vi "Get GUID.vi"(8 "error in (no error)":errorcluster) -> (0 "error out":errorcluster, 3 "GUID":string)   [LabVIEW 2013]
uses:
  <vilib>/registry/registry.llb/Registry RtKey.ctl
  <vilib>/registry/registry.llb/Registry SAM.ctl
  <vilib>/registry/registry.llb/Registry View.ctl
  <vilib>/registry/registry.llb/Read Registry Value Simple STR.vi
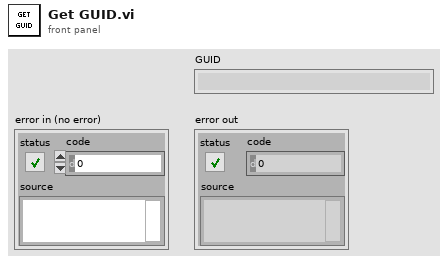
[diagram p1: front panel]
types:
  T1 = typedef "Registry SAM.ctl" = enum32{"KEY_QUERY_VALUE", "KEY_SET_VALUE", "KEY_CREATE_SUB_KEY", "KEY_ENUMERATE_SUB_KEYS", "KEY_NOTIFY", "KEY_CREATE_LINK", "KEY_READ", "KEY_WRITE", "KEY_ALL_ACCESS", "KEY_READ | KEY_WRITE"}
  T2 = typedef "Registry RtKey.ctl" = enum32{"HKEY_CLASSES_ROOT", "HKEY_CURRENT_USER", "HKEY_LOCAL_MACHINE", "HKEY_USERS", "HKEY_PERFORMANCE_DATA", "HKEY_CURRENT_CONFIG", "HKEY_DYN_DATA"}
  T3 = typedef "Registry View.ctl" = u16
  T4 = typedef "Registry refnum.ctl" = refnum<k1>
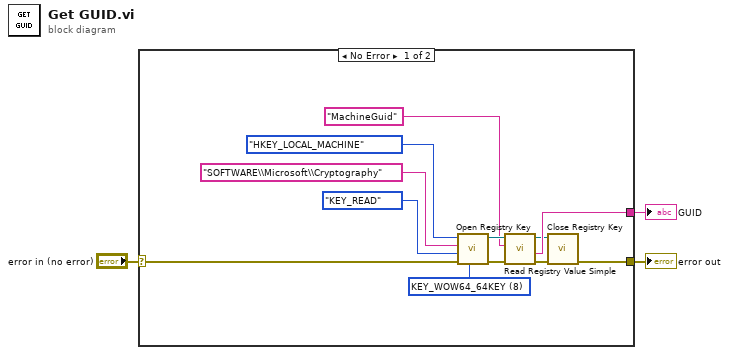
[diagram p0: block diagram]
diagram:
  n1 = case shown="No Error" "error in (no error)" {
    selector: "error in (no error)" -> [w15 w16]
    tunnel: [w14 w16] -> w2
    tunnel: [w13 _] -> w1
    frame No Error {
      w4 = T3 8 items=["Default"=0, "KEY_WOW64_64KEY"=8, "KEY_WOW64_32KEY"=9] ("registry view")
      n2 = call <vilib>:"Open Registry Key.vi"("registry view"=w4, "error in (no error)"=w15, "security access mask (KEY_READ | KEY_WRITE)"=Registry_SAM."KEY_READ", "subkey"="SOFTWARE\\Microsoft\\Cryptography", "root key (HKEY_LOCAL_MACHINE)"=Registry_RtKey."HKEY_LOCAL_MACHINE") -> ("error out"=w8:errorcluster, "refnum out"=w9:T4)  [unwired: 5 in]
      n3 = call-poly <vilib>:"Read Registry Value Simple.vi"("error in (no error)"=w8, "value"="MachineGuid", "refnum"=w9) -> ("error out"=w6:errorcluster, "String/Binary data"=w13:string, "refnum out"=w7:T4)  [unwired: 3 in, 1 out]
      n4 = call <vilib>:"Close Registry Key.vi"("error in (no error)"=w6, "refnum"=w7) -> ("error out"=w14:errorcluster)  [unwired: 5 in]
    }
    frame Error {
    }
  }
  "GUID" <- w1
  "error out" <- w2
